vi "006 System Gloabl Read&Write.vi"(8 "error in (no error)":errorcluster caption="Error In", 11 "RW":enum16{"Read", "Write"}(ring)) -> (0 "error out":errorcluster caption="Error Out", 1 "Config Path":path, 2 "Root Path":path, 3 "Project":string)   [LabVIEW 2020]
uses:
  006 System Gloabl.vi
  <vilib>/Utility/config.llb/Read Key (String).vi
  <vilib>/Utility/config.llb/Write Key (String).vi
  <vilib>/Utility/config.llb/NI_LVConfig.lvlib
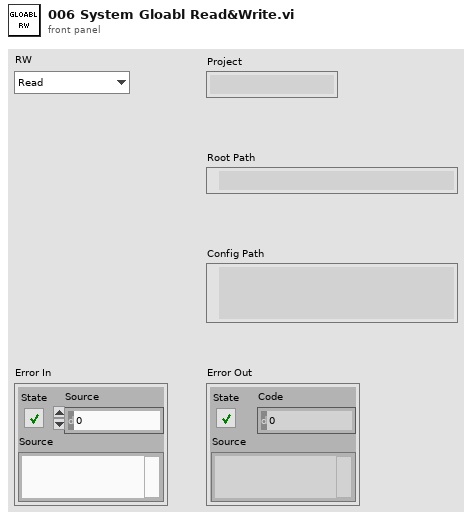
[diagram p1: front panel]
types:
  T1 = typedef "NI_LVConfig.lvlib/Config Data RefNum.ctl" = refnum<k1>
  T2 = enum32{"invalid app kind", "Development System", "Run Time System", "Student Edition", "Embedded LabVIEW", "Evaluation", "Custom"}
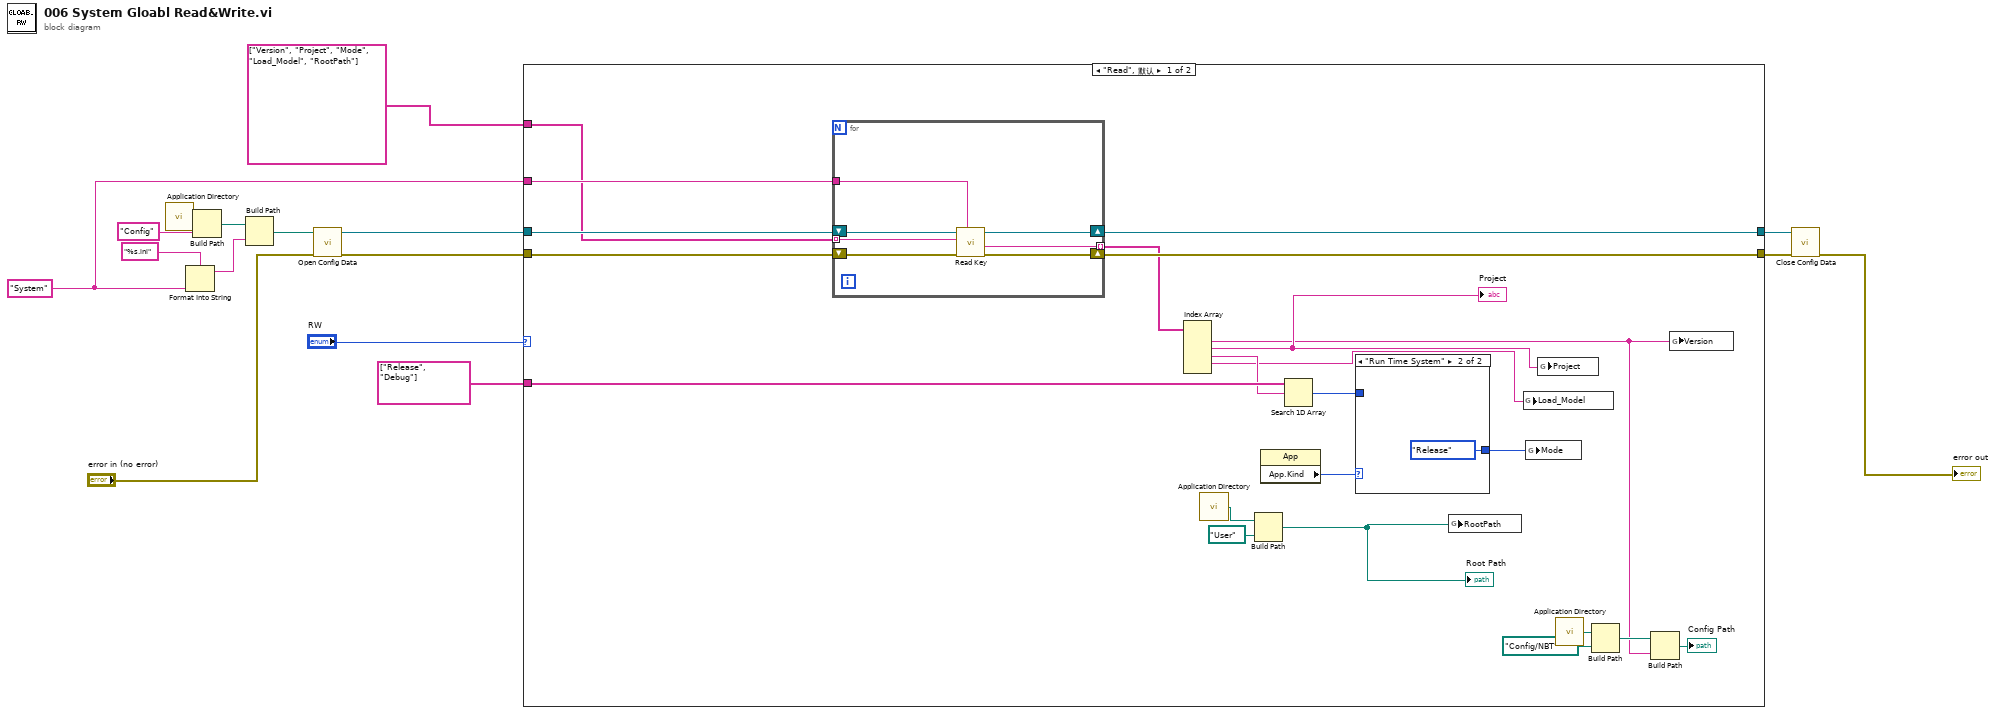
[diagram p0: block diagram]
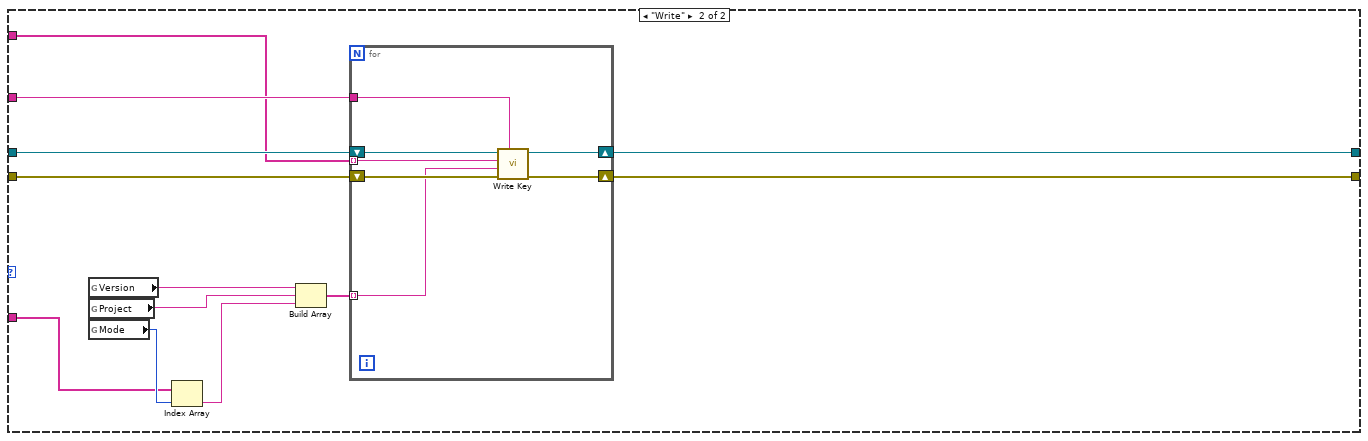
[diagram p3: hidden frame]
diagram:
  w5 = "System"
  n1 = call <vilib>:"Application Directory.vi"() -> ("Application Directory"=w16:path)
  n2 = Format Into String(format string="%s.ini" ("格式字符串"), w5) -> (resulting string=w12:string)  [unwired: 2 in, 1 out]
  n3 = Build Path(base path=w16, name or relative path="Config") -> (appended path=w14:path)
  n4 = Build Path(base path=w14, name or relative path=w12) -> (appended path=w11:path)
  n5 = call <vilib>:"Open Config Data.vi"("error in (no error)"="error in (no error)", "configuration file path"=w11) -> ("error out"=w7:errorcluster, "refnum"=w10:T1)  [unwired: 7 in, 1 out]
  n6 = case shown="\"Read\", 默认" "RW" {
    tunnel: w10 -> [w38 w59]
    tunnel: [w37 w58] -> w9
    tunnel: w7 -> [w36 w57]
    tunnel: [w35 w56] -> w6
    tunnel: w5 -> [w34 w55]
    tunnel: string[] ["Version", "Project", "Mode", "Load_Model", "RootPath"] -> [w33 w54]
    tunnel: string[] ["Release", "Debug"] -> [w31 w48]
    frame "Read", Default {
      n7 = for {
        tunnel: w34 -> [w43]
        shift-right: [w46] -> w37
        shift-left: w38 -> [w47]
        shift-right: [w44] -> w35
        shift-left: w36 -> [w45]
        tunnel: w33 -> [w42] mode=indexing
        tunnel: [w41] -> w32 mode=indexing
        n8 = call-poly <vilib>:"Read Key.vi"("section"=w43, "error in (no error)"=w45, "key"=w42, "refnum"=w47) -> ("error out"=w44:errorcluster, "value"=w41:string, "refnum out"=w46:T1)  [unwired: 4 in, 1 out]
      }
      n9 = Index Array(array=w32) -> (element #1=w21:string, element #2=w29:string, element #3=w30:string, element #4=w25:string)  [unwired: 5 in, 1 out]
      "Project" <- w29
      n10 = call <vilib>:"Application Directory.vi"() -> ("Application Directory"=w19:path)
      n11 = Build Path(base path=w19, name or relative path=path "User" ("名称或相对路径")) -> (appended path=w17:path)
      "Root Path" <- w17
      n12 = property class="App"() -> ("App.Kind"=w28:T2)  [unwired: 2 in, 2 out]
      n13 = Search 1D Array(1D array=w31, element=w30) -> (index of element=w26:i32)  [unwired: 1 in]
      n14 = case shown="\"Run Time System\"" w28 {
        tunnel: [w39 enum16{"Release", "Debug"}."Release" ("Mode")] -> w27
        tunnel: w26 -> [w39 _]
        frame "invalid app kind", Default {
        }
        frame "Run Time System" {
        }
      }
      n15 = global write "006 System Gloabl.vi" "RootPath"(w17) -> ()
      n16 = global write "006 System Gloabl.vi" "Load_Model"(w25) -> ()
      n17 = global write "006 System Gloabl.vi" "Mode"(w27) -> ()
      n18 = global write "006 System Gloabl.vi" "Project"(w29) -> ()
      n19 = call <vilib>:"Application Directory.vi"() -> ("Application Directory"=w24:path)
      n20 = Build Path(base path=w24, name or relative path=path "Config/NBT" ("名称或相对路径")) -> (appended path=w23:path)
      n21 = Build Path(base path=w23, name or relative path=w21) -> (appended path=→"Config Path":path)
      n22 = global write "006 System Gloabl.vi" "Version"(w21) -> ()
    }
    frame "Write" {
      n23 = global read "006 System Gloabl.vi" "Version"() -> (w51:string)
      n24 = global read "006 System Gloabl.vi" "Project"() -> (w52:string)
      n25 = global read "006 System Gloabl.vi" "Mode"() -> (w50:enum16{"Release", "Debug"})
      n26 = Index Array(array=w48, index=w50) -> (element=w53:string)
      n27 = Build Array(w51, w52, w53) -> (w49:string[])
      n28 = for {
        tunnel: w55 -> [w62]
        tunnel: w54 -> [w61] mode=indexing
        shift-right: [w65] -> w58
        shift-left: w59 -> [w66]
        shift-right: [w63] -> w56
        shift-left: w57 -> [w64]
        tunnel: w49 -> [w60] mode=indexing
        n29 = call-poly <vilib>:"Write Key.vi"("section"=w62, "error in (no error)"=w64, "value"=w60, "key"=w61, "refnum"=w66) -> ("error out"=w63:errorcluster, "refnum out"=w65:T1)  [unwired: 4 in, 1 out]
      }
    }
  }
  n30 = call <vilib>:"Close Config Data.vi"("error in (no error)"=w6, "refnum"=w9) -> ("error out"=→"error out":errorcluster)  [unwired: 8 in, 1 out]
